vi "Line_FGV.vi"(8 "error in (no error)":errorcluster, 9 "Message Data":variant, 11 "Message":string) -> (0 "error out":errorcluster, 1 "Message Data 2":variant, 3 "Message 2":string)   [LabVIEW 2016]
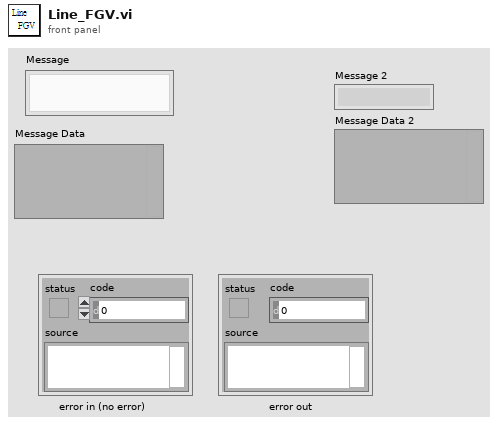
[diagram p1: front panel]
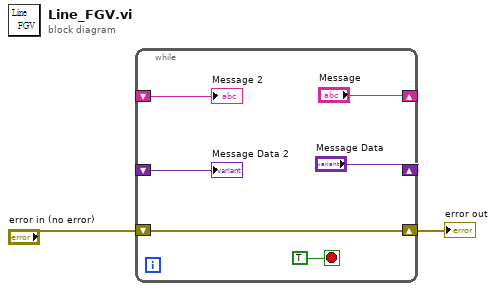
[diagram p0: block diagram]
diagram:
  n1 = while {
    shift-right: ["Message"] -> _
    shift-left: _ -> [w5]
    shift-right: ["Message Data"] -> _
    shift-left: _ -> [w4]
    shift-right: [w3] -> w1
    shift-left: "error in (no error)" -> [w3]
    stop <- TRUE stop-if-true
    "Message 2" <- w5
    "Message Data 2" <- w4
  }
  "error out" <- w1
